vi "Perform Action.vi"(8 "error in (no error)":errorcluster, 10 "Input":variant, 11 "Fetch Waveforms CFG in":refnum<class "Fetch Waveforms CFG.lvclass">) -> (0 "error out":errorcluster, 2 "Output":variant, 3 "Fetch Waveforms CFG out":refnum<class "Fetch Waveforms CFG.lvclass">)   [LabVIEW 2023, in "Thermometer Simulated CFGs.lvlib" / "Fetch Waveforms CFG.lvclass"]
uses:
  Fetch Waveforms CFG.lvclass
  Fetch Waveforms CFG.lvclass/Fetch Waveforms CFG.ctl
  <vilib>/measure/NI_MABase.lvlib
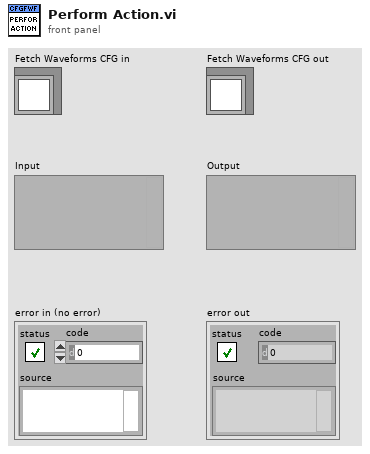
[diagram p1: front panel]
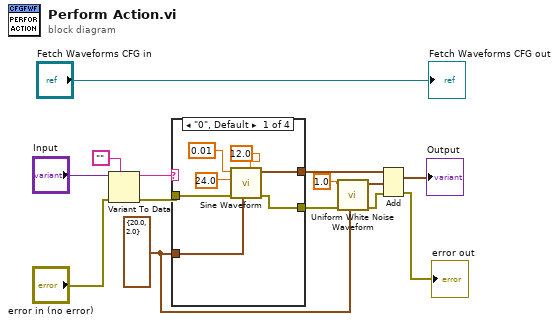
[diagram p0: block diagram]
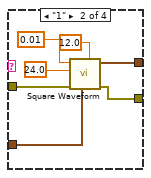
[diagram p2: hidden frame]
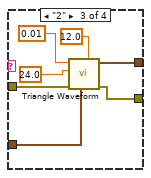
[diagram p3: hidden frame]
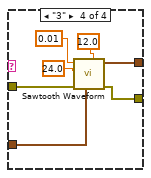
[diagram p4: hidden frame]
diagram:
  w1 = cluster{"Fs":dbl, "#s":dbl} {"Fs"=20.0, "#s"=2.0} ("sampling info")
  n1 = Variant To Data(error in="error in (no error)", type="", Variant="Input") -> (data=w7:string, error out=w8:errorcluster)
  n2 = case shown="\"0\", Default" w7 {
    tunnel: [w21 w27 w34 w42] -> w13
    tunnel: w8 -> [w20 w28 w35 w41]
    tunnel: [w19 w26 w33 w40] -> w10
    tunnel: w1 -> [w15 w22 w32 w36]
    frame "0", Default {
      n3 = call <vilib>:"Sine Waveform.vi"("offset"=12.0, "sampling info"=w15, "error in (no error)"=w20, "amplitude"=24.0, "frequency"=0.01) -> ("error out"=w19:errorcluster, "signal out"=w21:waveform(dbl))  [unwired: 5 in]
    }
    frame "1" {
      n4 = call <vilib>:"Square Waveform.vi"("offset"=12.0, "sampling info"=w22, "error in (no error)"=w28, "amplitude"=24.0, "frequency"=0.01) -> ("error out"=w26:errorcluster, "signal out"=w27:waveform(dbl))  [unwired: 5 in]
    }
    frame "2" {
      n5 = call <vilib>:"Triangle Waveform.vi"("offset"=12.0, "sampling info"=w32, "error in (no error)"=w35, "amplitude"=24.0, "frequency"=0.01) -> ("error out"=w33:errorcluster, "signal out"=w34:waveform(dbl))  [unwired: 5 in]
    }
    frame "3" {
      n6 = call <vilib>:"Sawtooth Waveform.vi"("offset"=12.0, "sampling info"=w36, "error in (no error)"=w41, "amplitude"=24.0, "frequency"=0.01) -> ("error out"=w40:errorcluster, "signal out"=w42:waveform(dbl))  [unwired: 5 in]
    }
  }
  n7 = call <vilib>:"Uniform White Noise Waveform.vi"("sampling info"=w1, "error in (no error)"=w10, "amplitude"=1.0) -> ("error out"=w9:errorcluster, "signal out"=w12:waveform(dbl))  [unwired: 7 in]
  n8 = Add(1:w12, 2:w13, 4:w9) -> (0:→"Output":waveform(dbl), 3:→"error out":errorcluster)
  "Fetch Waveforms CFG out" <- "Fetch Waveforms CFG in"
